vi "Traverse comms checker.vi"() -> ()   [LabVIEW 2022 SP3]
uses:
  ~subVIs/DriveProperties.ctl
  ~subVIs/DriveStaticConfig.ctl
  ~subVIs/AxisConfigCluster.ctl
panel:
  out "Hz":dbl
  in  "Matched Configurations":T1[](array[typedef])=[{"Channel Properties"={"Channel Name"="EnFlo_Trav1:Motor:X", "Vel. Default"=5.775, "Acc. Default"=10.0, "Vel. Max"=8.0, "Vel. Min"=0.1, "Acc. Max"=10.0, "Acc. Min"=0.5, "Pulses/unit"=-170.665, "Address"=4, "Pulse Offset"=-8047, "Pos Tolerance"=0.01, "Pulses/rev"=2048.0, "Backlash/Eng units"=-3.0, "Current Pos"=-0.0, "Ch Status"=enum."Active", "Port Name"="COM9", "Axis Transform mode"="", "Metadata Ch Name"="EnFlo_Tunnel:Trav1 Pos:X", "Type"="MCode"}, "Static Drive Configuration"={"Correction Gain % (CG)"=1, "Dead Band (DB)"=100, "Dead Band Window (DW)"=350, "Encoder Resolution (ER)"=4000, "Step Mode  (FSB)"=1, "Position Maintenance (FSC)"=0, "Stop on Stall (FSD)"=1, "Activate OP1 on stall (FSE)"=0, "Stop on Trigger 3 (FSF)"=1, "OP2 in Deadband (FSG)"=0, "Stall Detect (FSH)"=1, "Limit Disable (LD)"=0, "Motor Resolution (MR)"=enum."25000", "Limit Switch Sense (OSA)"=0, "Home Position (OSB)"=1, "Home Switch Sense (OSC)"=0, "Encoder Z for Home (OSD)"=1, "Reference edge of Home (OSH)"=0, "RS232 Echo Control (SSA)"=0, "Buffer at Limit (SSG)"=1, "Buffer at Stop (SSH)"=1, "Indexer Mode  (FSA)"=1, "Type"="MCode", "ConfigString"="EM=0;DB=5;ES=2;HC=5;HT=500;JE=1;LM=6;MS=256;PM=0;RC=100;S1=6,0,0;S2=1,0,1;S3=5,0,0;S4=18,0,0;SF=200;SM=0;VI=40;S;", "De Power Motor"=enum."TRUE"}}, {"Channel Properties"={"Channel Name"="EnFlo_Trav1:Motor:Y", "Vel. Default"=7.349999, "Acc. Default"=4.2, "Vel. Max"=100.0, "Vel. Min"=0.1, "Acc. Max"=100.0, "Acc. Min"=0.2, "Pulses/unit"=-292.44, "Address"=6, "Pulse Offset"=-201112, "Pos Tolerance"=0.01, "Pulses/rev"=2048.0, "Backlash/Eng units"=2.0, "Current Pos"=125.00342, "Ch Status"=enum."Active", "Port Name"="COM9", "Axis Transform mode"="", "Metadata Ch Name"="EnFlo_Tunnel:Trav1 Pos:Y", "Type"="MCode"}, "Static Drive Configuration"={"Correction Gain % (CG)"=1, "Dead Band (DB)"=10, "Dead Band Window (DW)"=30, "Encoder Resolution (ER)"=2048, "Step Mode  (FSB)"=1, "Position Maintenance (FSC)"=0, "Stop on Stall (FSD)"=1, "Activate OP1 on stall (FSE)"=0, "Stop on Trigger 3 (FSF)"=1, "OP2 in Deadband (FSG)"=0, "Stall Detect (FSH)"=1, "Limit Disable (LD)"=3, "Motor Resolution (MR)"=enum."25000", "Limit Switch Sense (OSA)"=0, "Home Position (OSB)"=1, "Home Switch Sense (OSC)"=0, "Encoder Z for Home (OSD)"=1, "Reference edge of Home (OSH)"=0, "RS232 Echo Control (SSA)"=0, "Buffer at Limit (SSG)"=1, "Buffer at Stop (SSH)"=1, "Indexer Mode  (FSA)"=1, "Type"="MCode", "ConfigString"="EM=0;DB=5;ES=2;HC=5;HT=500;JE=1;LM=6;MS=256;PM=0;RC=20;S1=6,0,0;S2=1,0,1;S3=5,0,0;S4=18,0,0;SF=200;SM=0;VI=40;S;", "De Power Motor"=enum."TRUE"}}, {"Channel Properties"={"Channel Name"="EnFlo_Trav1:Motor:Z", "Vel. Default"=20.0, "Acc. Default"=20.0, "Vel. Max"=40.0, "Vel. Min"=0.1, "Acc. Max"=35.0, "Acc. Min"=0.2, "Pulses/unit"=-2048.0, "Address"=8, "Pulse Offset"=-1517978, "Pos Tolerance"=0.01, "Pulses/rev"=2048.0, "Backlash/Eng units"=2.0, "Current Pos"=700.0, "Ch Status"=enum."Active", "Port Name"="COM9", "Axis Transform mode"="", "Metadata Ch Name"="EnFlo_Tunnel:Trav1 Pos:Z", "Type"="MCode"}, "Static Drive Configuration"={"Correction Gain % (CG)"=1, "Dead Band (DB)"=10, "Dead Band Window (DW)"=30, "Encoder Resolution (ER)"=2048, "Step Mode  (FSB)"=1, "Position Maintenance (FSC)"=0, "Stop on Stall (FSD)"=1, "Activate OP1 on stall (FSE)"=0, "Stop on Trigger 3 (FSF)"=1, "OP2 in Deadband (FSG)"=0, "Stall Detect (FSH)"=1, "Limit Disable (LD)"=0, "Motor Resolution (MR)"=enum."25000", "Limit Switch Sense (OSA)"=0, "Home Position (OSB)"=1, "Home Switch Sense (OSC)"=0, "Encoder Z for Home (OSD)"=1, "Reference edge of Home (OSH)"=0, "RS232 Echo Control (SSA)"=0, "Buffer at Limit (SSG)"=1, "Buffer at Stop (SSH)"=1, "Indexer Mode  (FSA)"=1, "Type"="MCode", "ConfigString"="EM=0;DB=5;ES=2;HC=5;HT=500;JE=1;LM=6;MS=256;PM=0;RC=50;S1=2,0,0;S2=1,0,1;S3=5,0,0;S4=18,0,0;SF=200;SM=0;VI=40;S;", "De Power Motor"=enum."TRUE"}}] {"Static Drive Configuration"."Indexer Mode  (FSA)" items=["Incremental", "Absolute"]; "Static Drive Configuration"."Buffer at Stop (SSH)" items=["Clear buffer", "Save and Continue"]; "Static Drive Configuration"."Buffer at Limit (SSG)" items=["Clear buffer", "Save and Continue"]; "Static Drive Configuration"."RS232 Echo Control (SSA)" items=["Echo ON", "Echo OFF"]; "Static Drive Configuration"."Reference edge of Home (OSH)" items=["CW", "CCW"]; "Static Drive Configuration"."Encoder Z for Home (OSD)" items=["Don't use", "Enable"]; "Static Drive Configuration"."Home Switch Sense (OSC)" items=["Normally Open", "Normally Closed"]; "Static Drive Configuration"."Home Position (OSB)" items=["Anywhere in Switch", "Edge of Switch"]; "Static Drive Configuration"."Limit Switch Sense (OSA)" items=["Normally Closed", "Normally Open"]; "Static Drive Configuration"."Limit Disable (LD)" items=["Both Enabled", "CW Disabled", "CCW Disabled", "Both Disabled"]; "Static Drive Configuration"."Stall Detect (FSH)" items=["Disable", "Enable"]; "Static Drive Configuration"."OP2 in Deadband (FSG)" items=["Don't Use", "ACTIVATE"]; "Static Drive Configuration"."Stop on Trigger 3 (FSF)" items=["Ignore", "STOP!"]; "Static Drive Configuration"."Activate OP1 on stall (FSE)" items=["Do not Activate", "ACTIVATE!"]; "Static Drive Configuration"."Stop on Stall (FSD)" items=["Continue", "STOP"]; "Static Drive Configuration"."Position Maintenance (FSC)" items=["Disabled", "Enabled"]; "Static Drive Configuration"."Step Mode  (FSB)" items=["Motor", "Encoder"]; "Static Drive Configuration"."Encoder Resolution (ER)" min=1 max=50000; "Static Drive Configuration"."Dead Band Window (DW)" min=0 max=999999999; "Static Drive Configuration"."Dead Band (DB)" min=0 max=999999999; "Static Drive Configuration"."Correction Gain % (CG)" items=["n/a", "12.5", "25", "37.5", "50", "62.5", "75", "87.5", "100"]; "Channel Properties"."Current Pos" format="%.2f"; "Channel Properties"."Backlash/Eng units" format="%.2f"; "Channel Properties"."Pulses/rev" format="%.2f"; "Channel Properties"."Pos Tolerance" format="%.2f"; "Channel Properties"."Pulses/unit" format="%.2f"; "Channel Properties"."Acc. Min" format="%.2f"; "Channel Properties"."Acc. Max" format="%.2f"; "Channel Properties"."Vel. Min" format="%.2f"; "Channel Properties"."Vel. Max" format="%.2f"; "Channel Properties"."Acc. Default" format="%.2f"; "Channel Properties"."Vel. Default" format="%.2f"}
  out "Numeric":i32
  in  "index":i32
  out "Waveform Chart 3":sgl(graph)
  out "Waveform Chart 2":sgl(graph)
  out "Waveform Chart":sgl(graph)
  in  "stop":bool
  in  "Recheck if Moved?":bool
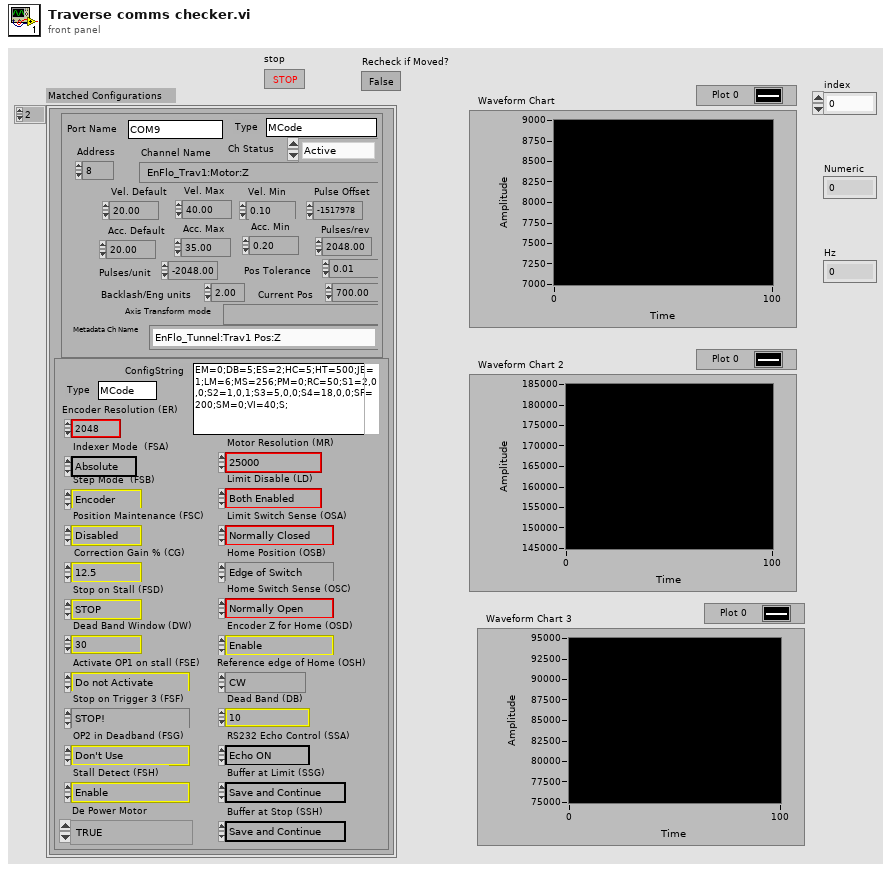
[diagram p1: front panel]
types:
  T1 = typedef "AxisConfigCluster.ctl" = cluster{"Channel Properties":T2, "Static Drive Configuration":T3}
  T2 = typedef "DriveProperties.ctl" = cluster{"Channel Name":string, "Vel. Default":sgl, "Acc. Default":sgl, "Vel. Max":sgl, "Vel. Min":sgl, "Acc. Max":sgl, "Acc. Min":sgl, "Pulses/unit":sgl, "Address":u8, "Pulse Offset":i32, "Pos Tolerance":sgl, "Pulses/rev":sgl, "Backlash/Eng units":sgl, "Current Pos":sgl, "Ch Status":enum16{"Active", "Offline", "Simulate"}, "Port Name":string, "Axis Transform mode":string, "Metadata Ch Name":string, "Type":string}
  T3 = typedef "DriveStaticConfig.ctl" = cluster{"Correction Gain % (CG)":u16, "Dead Band (DB)":i32, "Dead Band Window (DW)":i32, "Encoder Resolution (ER)":i32, "Step Mode  (FSB)":u16, "Position Maintenance (FSC)":u16, "Stop on Stall (FSD)":u16, "Activate OP1 on stall (FSE)":u16, "Stop on Trigger 3 (FSF)":u16, "OP2 in Deadband (FSG)":u16, "Stall Detect (FSH)":u16, "Limit Disable (LD)":u16, "Motor Resolution (MR)":enum16{"200", "400", "1000", "2000", "4000", "5000", "10000", "12800", "18000", "20000", "21600", "25000", "25400", "25600", "36000", "50000", "278528", "425984", "507904", "614400", "655360", "819200", "1024000"}, "Limit Switch Sense (OSA)":u16, "Home Position (OSB)":u16, "Home Switch Sense (OSC)":u16, "Encoder Z for Home (OSD)":u16, "Reference edge of Home (OSH)":u16, "RS232 Echo Control (SSA)":u16, "Buffer at Limit (SSG)":u16, "Buffer at Stop (SSH)":u16, "Indexer Mode  (FSA)":u16, "Type":string, "ConfigString":string, "De Power Motor":enum16{"TRUE", "FALSE"}}
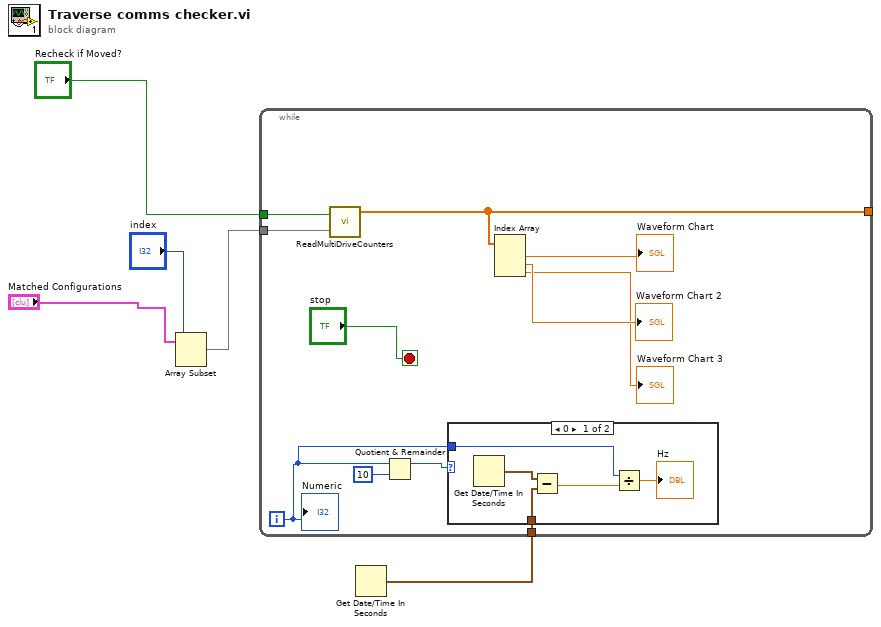
[diagram p0: block diagram]
diagram:
  n1 = Array Subset(array="Matched Configurations", index="index") -> (w3:T1[])  [unwired: 1 in]
  n2 = Get Date/Time In Seconds() -> (seconds since 1Jan1904=w1:timestamp)
  n3 = while {
    tunnel: w3 -> [w16]
    tunnel: "Recheck if Moved?" -> [w15]
    tunnel: [w13] -> _
    tunnel: w1 -> [w7]
    i -> [w6]
    stop <- "stop" stop-if-true
    n4 = call "ReadMultiDriveCounters.vi"("Recheck if Moved?"=w15, "Matched Configurations"=w16) -> ("Pulses"=w13:sgl[])  [unwired: 2 out]
    n5 = Quotient & Remainder(x=w6, y=10) -> (x-y*floor(x/y)=w8:i32)  [unwired: 1 out]
    n6 = case shown="0" w8 {
      tunnel: w7 -> [w20 _]
      tunnel: w6 -> [w19 _]
      frame 0 {
        n7 = Get Date/Time In Seconds() -> (seconds since 1Jan1904=w21:timestamp)
        n8 = Subtract(x=w21, y=w20) -> (x-y=w18:dbl)
        n9 = Divide(x=w19, y=w18) -> (x/y=→"Hz":dbl)
      }
      frame 1, Default {
      }
    }
    n10 = Index Array(array=w13) -> (element #1=→"Waveform Chart":sgl, element #2=→"Waveform Chart 2":sgl, element #3=→"Waveform Chart 3":sgl)  [unwired: 3 in]
    "Numeric" <- w6
  }
